vi "RT Test.vi"() -> ()   [LabVIEW 2016]
uses:
  Remote Terminal/TypeDefs/Command Configuration.ctl
  Remote Terminal/TypeDefs/Command Type.ctl
  1553 SubComponent/TypeDefs/Parameter Table Data.ctl
  1553 SubComponent/TypeDefs/Scaling Information.ctl
  Remote Terminal/TypeDefs/RT Configuration.ctl
  Remote Terminal/Remote Terminal.lvclass
  D:/SVN/Products/BCI-1553/Software/Development/2016/RealTime/1553 SubComponent/1553 SubComponent.lvclass
  1553 Board/1553 Board.lvclass
  1553 Component/1553 Component.lvclass
  1553 SubComponent/1553 SubComponent.lvclass
  Utilities/FPGA Interface/FPGA Interface.lvclass
panel:
  out "Scaled Data":dbl[][](array[numeric])
  out "Parameters":string[][](array[string])
  in  "stop":bool
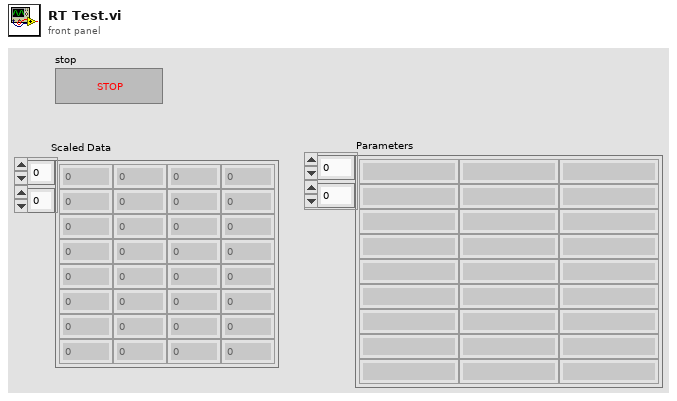
[diagram p1: front panel]
types:
  T1 = typedef "BCI-1553 API.lvlib/Remote Terminal.lvclass/RT Configuration.ctl" = cluster{"RT-RT TimeOut (us)":u8, "Inhibit Bus A":bool, "Inhibit Bus B":bool, "Broadcast CMD Invalid":bool, "UnDef MCs Invalid":bool, "Notice 2 Data Storage":bool, "SMCP":bool, "Temp RX Buffer":bool, "Alt BIT Enable":bool, "Auto Bus Shutdown":bool, "MC 17 Sync":u8, "MC 16 SR Reset":bool, "MC 8 Reset":bool}
  T2 = typedef "BCI-1553 API.lvlib/1553 SubComponent.lvclass/Parameter Table Data.ctl" = cluster{"Parameter Name":string, "Base Word":u16, "Address":u16, "Value":u64, "Mask":u16[], "Scaling Info":T3}
  T3 = typedef "BCI-1553 API.lvlib/1553 SubComponent.lvclass/Scaling Information.ctl" = cluster{"Bit Offset":i32, "Bit Count":i32, "LSB Resolution":dbl, "2's Complement":bool, "Big Endian":bool, "Sign Bit":bool}
  T4 = typedef "BCI-1553 API.lvlib/Remote Terminal.lvclass/Command Type.ctl" = enum16{"Transmit", "Receive", "Mode Code Tx", "Mode Code Rx"}
  T5 = typedef "BCI-1553 API.lvlib/Remote Terminal.lvclass/Command Configuration.ctl" = cluster{"Command Type":T4, "Mode Code ID (1-32)":u16, "SubAddress (1-30)":u16, "Word Count (1-32)":u16, "Illegal Command":bool, "Broadcast":bool, "Data":u16[], "Data Fields":T2[]}
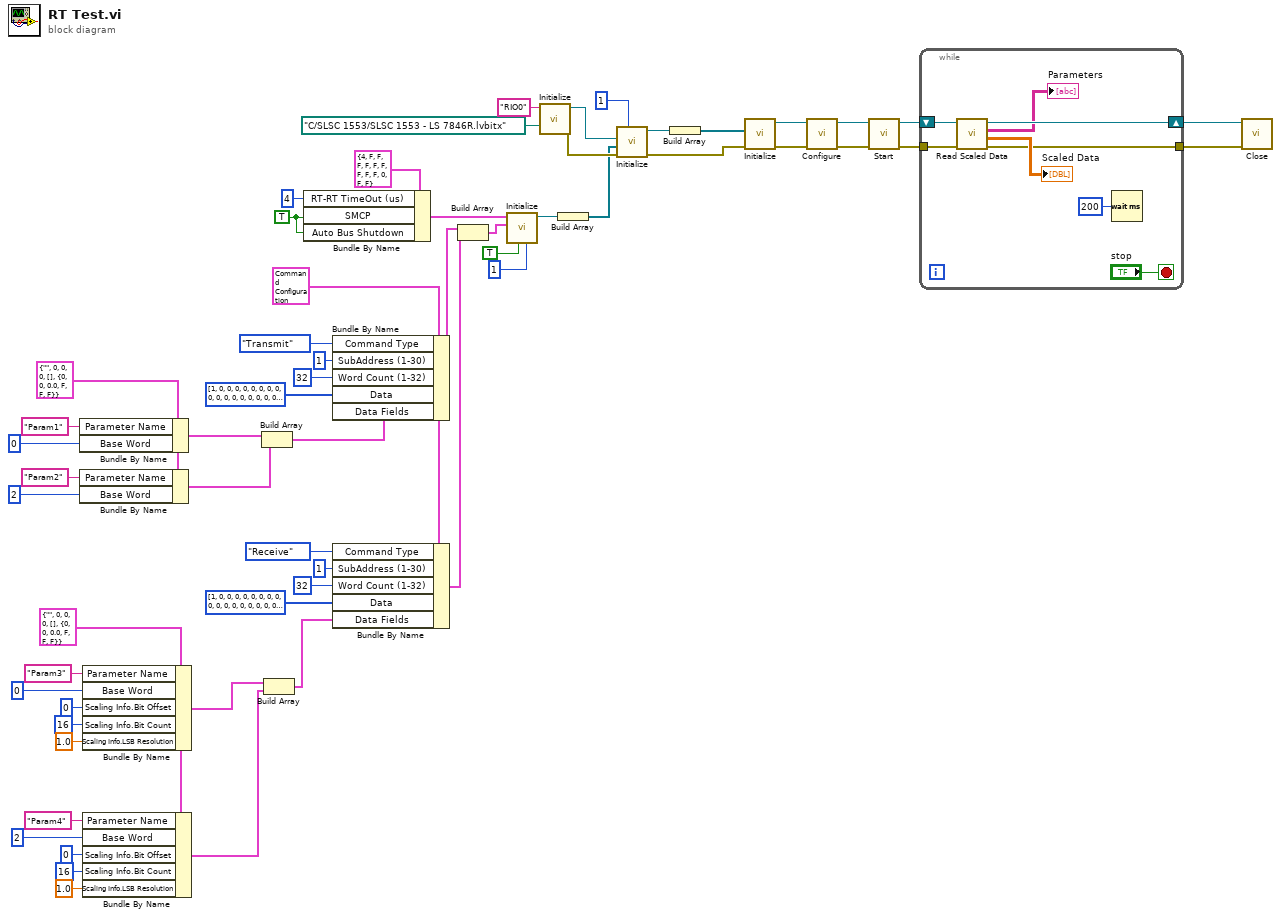
[diagram p0: block diagram]
diagram:
  w8 = TRUE ("SMCP")
  w17 = T2 {"Parameter Name"="", "Base Word"=0, "Address"=0, "Value"=0, "Mask"=[], "Scaling Info"={"Bit Offset"=0, "Bit Count"=0, "LSB Resolution"=0.0, "2's Complement"=FALSE, "Big Endian"=FALSE, "Sign Bit"=FALSE}} ("Parameter Table Data")
  w27 = T2 {"Parameter Name"="", "Base Word"=0, "Address"=0, "Value"=0, "Mask"=[], "Scaling Info"={"Bit Offset"=0, "Bit Count"=0, "LSB Resolution"=0.0, "2's Complement"=FALSE, "Big Endian"=FALSE, "Sign Bit"=FALSE}} ("Parameter Table Data")
  w22 = T5 {"Command Type"=enum."Transmit", "Mode Code ID (1-32)"=0, "SubAddress (1-30)"=1, "Word Count (1-32)"=32, "Illegal Command"=FALSE, "Broadcast"=FALSE, "Data"=[1, 0, 0, 0, 0, 0, 0, 0, 0, 0, 0, 0, 0, 0, 0, 0, 0, 0, 0, 0, 43690, 0, 0, 0, 0, 0, 0, 0, 0, 0, 0, 65535], "Data Fields"=[{"Parameter Name"="P1", "Base Word"=0, "Address"=0, "Value"=0, "Mask"=[], "Scaling Info"={"Bit Offset"=0, "Bit Count"=0, "LSB Resolution"=0.0, "2's Complement"=FALSE, "Big Endian"=FALSE, "Sign Bit"=FALSE}}]} ("CMD Configuration")
  n1 = Bundle By Name(cluster=w27, "Parameter Name"="Param1", "Base Word"=u16 0) -> (w29:T2)
  n2 = Bundle By Name(cluster=w27, "Parameter Name"="Param2", "Base Word"=u16 2) -> (w28:T2)
  n3 = Bundle By Name(cluster=w17, "Parameter Name"="Param3", "Base Word"=u16 0, "Scaling Info.Bit Offset"=0, "Scaling Info.Bit Count"=16, "Scaling Info.LSB Resolution"=1.0) -> (w16:T2)
  n4 = Bundle By Name(cluster=w17, "Parameter Name"="Param4", "Base Word"=u16 2, "Scaling Info.Bit Offset"=0, "Scaling Info.Bit Count"=16, "Scaling Info.LSB Resolution"=1.0) -> (w15:T2)
  n5 = Build Array(w29, w28) -> (w30:T2[])
  n6 = Build Array(w16, w15) -> (w14:T2[])
  n7 = Bundle By Name(cluster=T1 {"RT-RT TimeOut (us)"=4, "Inhibit Bus A"=FALSE, "Inhibit Bus B"=FALSE, "Broadcast CMD Invalid"=FALSE, "UnDef MCs Invalid"=FALSE, "Notice 2 Data Storage"=FALSE, "SMCP"=FALSE, "Temp RX Buffer"=FALSE, "Alt BIT Enable"=FALSE, "Auto Bus Shutdown"=FALSE, "MC 17 Sync"=0, "MC 16 SR Reset"=FALSE, "MC 8 Reset"=FALSE} ("RT Configuration"), "RT-RT TimeOut (us)"=u8 4, "SMCP"=w8, "Auto Bus Shutdown"=w8) -> (w7:T1)
  n8 = Bundle By Name(cluster=w22, "Command Type"=Command_Type."Transmit", "SubAddress (1-30)"=u16 1, "Word Count (1-32)"=u16 32, "Data"=u16[] [1, 0, 0, 0, 0, 0, 0, 0, 0, 0, 0, 0, 0, 0, 0, 0, 0, 0, 0, 0, 0, 0, 0, 0, 0, 0, 0, 0, 0, 0, 0, 65535], "Data Fields"=w30) -> (w13:T5)
  n9 = Bundle By Name(cluster=w22, "Command Type"=Command_Type."Receive", "SubAddress (1-30)"=u16 1, "Word Count (1-32)"=u16 32, "Data"=u16[] [1, 0, 0, 0, 0, 0, 0, 0, 0, 0, 0, 0, 0, 0, 0, 0, 0, 0, 0, 0, 0, 0, 0, 0, 0, 0, 0, 0, 0, 0, 0, 65535], "Data Fields"=w14) -> (w12:T5)
  n10 = Build Array(w13, w12) -> (w11:T5[])
  n11 = call "Initialize.vi"("RT Address (0-30)"=u8 1, "RT 1?"=TRUE, "Commands"=w11, "RT Configuration"=w7) -> ("Remote Terminal out"=w40:refnum<class "Remote Terminal.lvclass">)  [unwired: 6 in, 1 out]
  n12 = call "Initialize.vi"("Bitfile path"=path "C:/SLSC 1553/SLSC 1553 - LS 7846R.lvbitx", "Device address"="RIO0") -> ("error out"=w43:errorcluster, "FPGA Interface out"=w44:refnum<class "FPGA Interface.lvclass">)  [unwired: 8 in]
  n13 = Build Array(w40) -> (w39:refnum<class "Remote Terminal.lvclass">[])
  n14 = call "Initialize.vi"("Component ID (1-8)"=u8 1, "error in (no error)"=w43, "SubComponents"=w39, "FPGA Interface"=w44) -> ("error out"=w49:errorcluster, "1553 Component out"=w50:refnum<class "1553 Component.lvclass">)  [unwired: 6 in]
  n15 = Build Array(w50) -> (w48:refnum<class "1553 Component.lvclass">[])
  n16 = call "Initialize.vi"("error in (no error)"=w49, "Components"=w48) -> ("error out"=w55:errorcluster, "1553 Board out"=w58:refnum<class "1553 Board.lvclass">)  [unwired: 8 in]
  n17 = call-dynamic "Configure.vi"("error in (no error)"=w55, "1553 Board in"=w58) -> ("error out"=w56:errorcluster, "1553 Board out"=w57:refnum<class "1553 Board.lvclass">)  [unwired: 8 in]
  n18 = call-dynamic "Start.vi"("error in (no error)"=w56, "1553 Board in"=w57) -> ("error out"=w53:errorcluster, "1553 Board out"=w54:refnum<class "1553 Board.lvclass">)  [unwired: 8 in]
  n19 = while {
    shift-right: [w62] -> w52
    shift-left: w54 -> [w64]
    tunnel: w53 -> [w63]
    tunnel: [w59] -> w51
    stop <- "stop" stop-if-true
    n20 = call-dynamic "Read Scaled Data.vi"("error in (no error)"=w63, "1553 Board in"=w64) -> ("error out"=w59:errorcluster, "Scaled Data"=→"Scaled Data":dbl[][], "Parameters"=→"Parameters":string[][], "1553 Board out"=w62:refnum<class "1553 Board.lvclass">)  [unwired: 6 in]
    n21 = Wait (ms)(milliseconds to wait=u32 200) -> ()  [unwired: 1 out]
  }
  n22 = call-dynamic "Close.vi"("error in (no error)"=w51, "1553 Board in"=w52) -> ()  [unwired: 9 in, 1 out]
